vi "send.vi"(8 "error in (no error)":errorcluster, 11 "obj in":refnum<class "RequestBuilder.lvclass">) -> (0 "error out":errorcluster, 2 "request":refnum<class "Request.lvclass">)   [LabVIEW 2020, in "reqwest.lvlib" / "RequestBuilder.lvclass"]
uses:
  RequestBuilder.lvclass
  Request/Request.lvclass
  Request/request_id.ctl
  RequestBuilder.lvclass/RequestBuilder.ctl
  lv_reqwest_64.dll
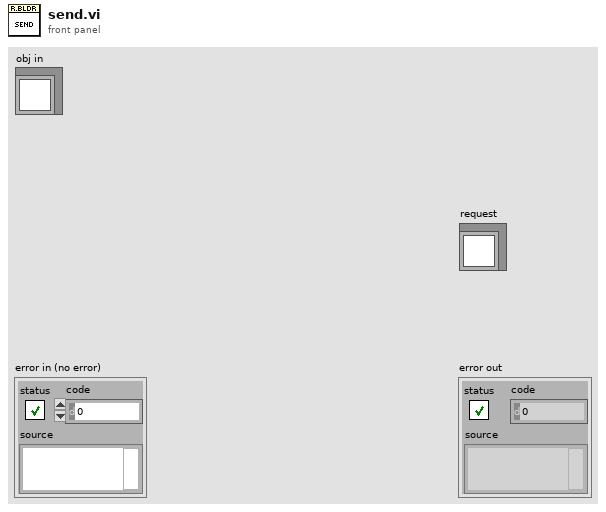
[diagram p1: front panel]
types:
  T1 = typedef "reqwest.lvlib/Request.lvclass/request_id.ctl" = u64
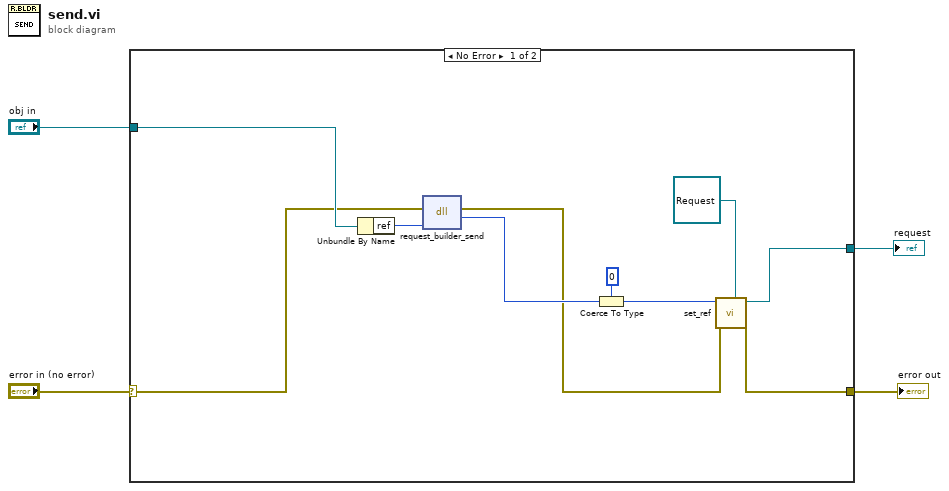
[diagram p0: block diagram]
diagram:
  n1 = case shown="No Error" "error in (no error)" {
    selector: "error in (no error)" -> [w13 w15]
    tunnel: "obj in" -> [w14 _]
    tunnel: [w7 w15] -> w2
    tunnel: [w9 _] -> w1
    frame No Error {
      n2 = Unbundle By Name(w14) -> ("ref"=w12:u64)
      n3 = dll-call lib="C:/Projects/reqwest-rs-labview/lv_src/lv_reqwest_*.*" fn="request_builder_send"(error in=w13, "request_builder_ref"=w12) -> (error out=w8:errorcluster, "request_id"=w10:u64)  [unwired: 3 in, 1 out]
      n4 = Coerce To Type(0:w10, 1:T1 0 ("request_id")) -> (2:w6:T1)
      n5 = call "set_ref.vi"("Request in"=refnum<class "Request.lvclass"> refnum, "error in (no error)"=w8, "request_id"=w6) -> ("error out"=w7:errorcluster, "Request out"=w9:refnum<class "Request.lvclass">)  [unwired: 7 in]
    }
    frame Error {
    }
  }
  "error out" <- w2
  "request" <- w1
